vi "destroy.vi"(8 "error in":errorcluster, 11 "Basic HTTP server in":refnum<class "Basic HTTP server.lvclass">) -> (0 "error out":errorcluster)   [LabVIEW 2013, in "Basic HTTP server.lvclass"]
uses:
  Basic HTTP server.lvclass
  Basic HTTP server.lvclass/Basic HTTP server.ctl
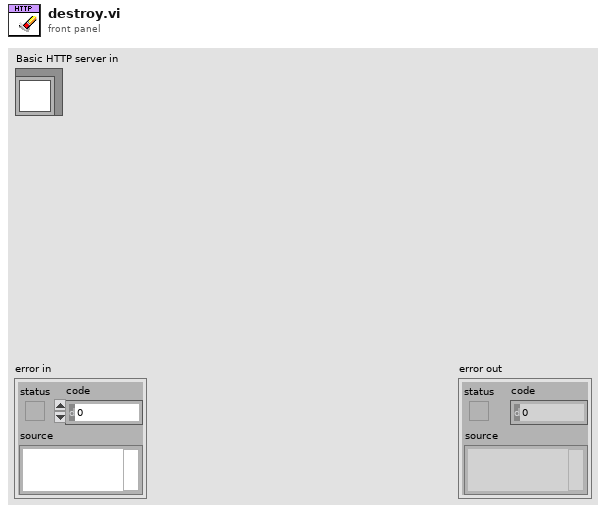
[diagram p1: front panel]
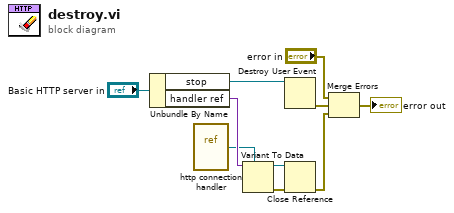
[diagram p0: block diagram]
diagram:
  n1 = Unbundle By Name("Basic HTTP server in") -> ("stop"=w7:refnum<user-event>, "handler ref"=w5:variant)
  n2 = vi-ref "http connection handler.vi"() -> (w4:refnum<vi>)
  n3 = Variant To Data(type=w4, Variant=w5) -> (data=w2:refnum<vi>, error out=w1:errorcluster)  [unwired: 1 in]
  n4 = Destroy User Event(user event=w7) -> (error out=w6:errorcluster)  [unwired: 1 in]
  n5 = Close Reference(reference=w2, error in (no error)=w1) -> (error out=w3:errorcluster)
  n6 = Merge Errors("error in", w6, w3) -> (→"error out":errorcluster)
